vi "Clear Arbitrary Waveform.vi"(7 "Arbitrary Waveform Name (0: USER1)":u16(ring) items=["USER1", "USER2", "USER3", "USER4"], 8 "error in (no error)":errorcluster, 11 "VISA resource name":refnum<visa-resource-name>) -> (0 "error out":errorcluster, 3 "VISA resource name out":refnum<visa-resource-name>)   [LabVIEW 2013, in "Tektronix AFG 3000 Series.lvlib"]
doc: "Removes a previously created arbitrary waveform from the function generator's memory.\n\n<B>Note:</B>\n\nAll arbitrary waveforms are stored in non-volatile memory and therefore will remain stored regardless of power-cycling, any waveforms that may contain sensitive material should be deleted after use."
uses:
  Tektronix AFG 3000 Series.lvlib
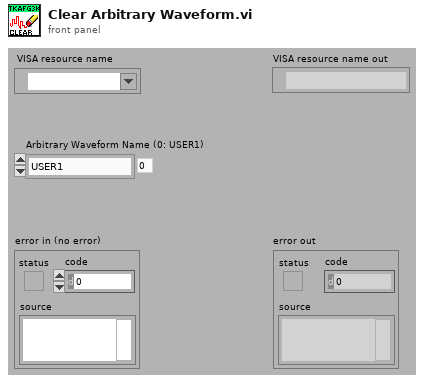
[diagram p1: front panel]
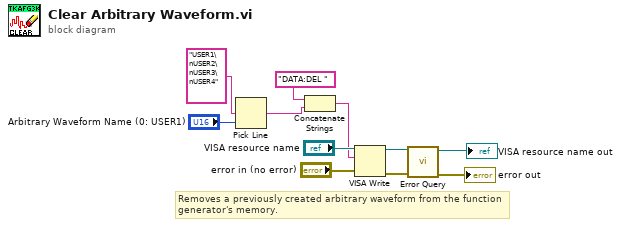
[diagram p0: block diagram]
diagram:
  # "Removes a previously created arbitrary waveform from the function \ngenerator's memory."
  n1 = Pick Line(multi-line string="USER1\nUSER2\nUSER3\nUSER4" ("string (\"\")"), line index="Arbitrary Waveform Name (0: USER1)") -> (output string=w3:string)  [unwired: 1 in]
  n2 = Concatenate Strings("DATA:DEL " ("string"), w3) -> (w8:string)
  n3 = VISA Write(VISA resource name="VISA resource name", write buffer=w8, error in (no error)="error in (no error)") -> (VISA resource name out=w7:refnum<visa-resource-name>, error out=w6:errorcluster)  [unwired: 1 out]
  n4 = call "Error Query.vi"("error in (no error)"=w6, "VISA resource name"=w7) -> ("error out"=→"error out":errorcluster, "VISA resource name out"=→"VISA resource name out":refnum<visa-resource-name>)  [unwired: 6 in, 2 out]
